vi "Check Firmware.vi"(10 "Actual":string, 11 "Cut-off":string) -> (3 "New Enough?":bool)   [LabVIEW 2013]
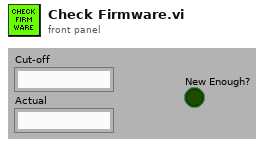
[diagram p1: front panel]
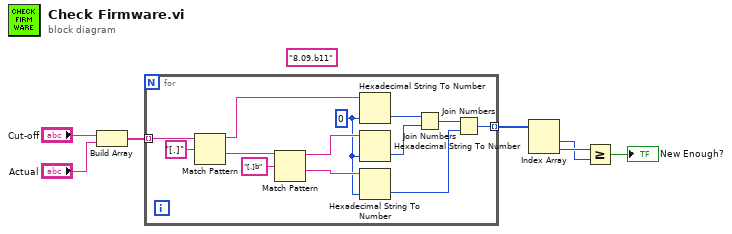
[diagram p0: block diagram]
diagram:
  (unwired) "8.09.b11" ("Firmware Version")
  n1 = Build Array("Cut-off", "Actual") -> (w5:string[])
  n2 = for {
    tunnel: w5 -> [w20] mode=indexing
    tunnel: [w9] -> w4 mode=indexing
    w8 = u8 0 ("default (0 U32)")
    n3 = Match Pattern(string=w20, regular expression="[.]") -> (before substring=w18:string, after substring=w16:string)  [unwired: 1 in, 2 out]
    n4 = Match Pattern(string=w16, regular expression="[.]b") -> (before substring=w15:string, after substring=w14:string)  [unwired: 1 in, 2 out]
    n5 = Hexadecimal String To Number(string=w18, default (0uL)=w8) -> (number=w13:u8)  [unwired: 1 in, 1 out]
    n6 = Hexadecimal String To Number(string=w15, default (0uL)=w8) -> (number=w12:u8)  [unwired: 1 in, 1 out]
    n7 = Hexadecimal String To Number(string=w14, default (0uL)=w8) -> (number=w10:u8)  [unwired: 1 in, 1 out]
    n8 = Join Numbers(hi=w13, lo=w12) -> ((hi.lo)=w11:u16)
    n9 = Join Numbers(hi=w11, lo=w10) -> ((hi.lo)=w9:u32)
  }
  n10 = Index Array(array=w4) -> (element #1=w2:u32, element #2=w3:u32)  [unwired: 2 in]
  n11 = Greater Or Equal?(x=w3, y=w2) -> (x >= y?=→"New Enough?":bool)
